vi "SortSchedules.vi"() -> (2 "arr out":string[](array[string]))   [LabVIEW 2020]
uses:
  7fad999f-577c-4f1c-871c-e9ed7f43c586.vi
  <vilib>/Array/Sort 2D Array - Pop Stack.vi
  <vilib>/Array/Sort 2D Array - Push Stack.vi
  7fad999f-577c-4f1c-871c-e9ed7f43c586.vi/269d4b3b-47f5-49e3-8884-44851e4dd9d5.vi
  7fad999f-577c-4f1c-871c-e9ed7f43c586.vi/6d99389c-673d-4efb-bf33-19b32bcf4cf8.vi
  Global variable.vi
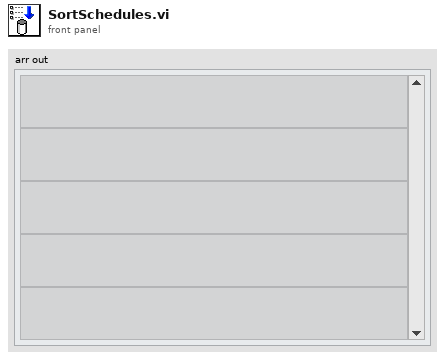
[diagram p1: front panel]
types:
  T1 = typedef "Schedule.ctl" = cluster{"Start time":timestamp, "Repeat":T2, "Action":T3}
  T2 = typedef "Repeat.ctl" = enum16{"None", "Every hour", "Every day", "Every week", "Every month"}
  T3 = typedef "Action.ctl" = u16
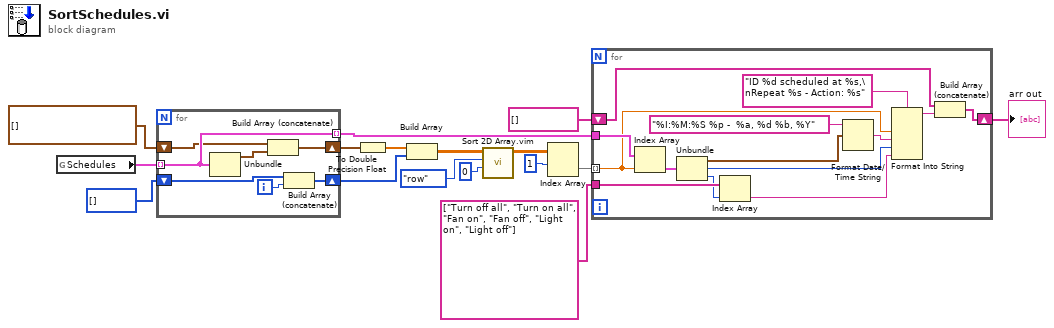
[diagram p0: block diagram]
diagram:
  n1 = global read "Global variable.vi" "Schedules"() -> (w1:T1[])
  n2 = for {
    tunnel: w1 -> [w22] mode=indexing
    shift-right: [w20] -> w10
    shift-left: timestamp[] [] -> [w18]
    tunnel: [w22] -> w16 mode=indexing
    shift-right: [w19] -> w11
    shift-left: i32[] [] -> [w17]
    i -> [w21]
    n3 = Unbundle(w22) -> ("Start time"=w23:timestamp)  [unwired: 2 out]
    n4 = Build Array (concatenate)(w18, w23) -> (w20:timestamp[])
    n5 = Build Array (concatenate)(w17, w21) -> (w19:i32[])
  }
  n6 = To Double Precision Float(number=w10) -> (double precision float=w9:dbl[])
  n7 = Build Array(w9, w11) -> (w8:dbl[][])
  n8 = call "Sort 2D Array.vim"("index"=0, "dimension to index (column)"=enum16{"column", "row"}."row", "2D array"=w8) -> ("sorted 2D array"=w5:dbl[][])  [unwired: 7 in, 1 out]
  n9 = Index Array(array=w5, index (row)=1) -> (element=w3:dbl[])  [unwired: 1 in]
  n10 = for {
    tunnel: w16 -> [w37]
    shift-right: [w31] -> w15
    shift-left: string[] [] -> [w25]
    tunnel: string[] ["Turn off all", "Turn on all", "Fan on", "Fan off", "Light on", "Light off"] -> [w27]
    tunnel: w3 -> [w28] mode=indexing
    n11 = Index Array(array=w37, index=w28) -> (element=w36:T1)
    n12 = Unbundle(w36) -> ("Start time"=w30:timestamp, "Repeat"=w29:T2, "Action"=w24:T3)
    n13 = Index Array(array=w27, index=w24) -> (element=w26:string)
    n14 = Format Date/Time String(time format string (%c)="%I:%M:%S %p -  %a, %d %b, %Y", seconds (now)=w30) -> (date/time string=w34:string)  [unwired: 1 in]
    n15 = Format Into String(format string="ID %d scheduled at %s,\nRepeat %s - Action: %s" ("FMT string"), w28, w34, w29, w26) -> (resulting string=w35:string)  [unwired: 2 in, 1 out]
    n16 = Build Array (concatenate)(w25, w35) -> (w31:string[])
  }
  "arr out" <- w15
